vi "GVmotor_get_Alarm.vi"(8 "error in (no error)":errorcluster, 10 "milliseconds to wait":u32=100, 11 "VISA resource name":refnum<visa-resource-name>) -> (0 "error out":errorcluster, 2 "Alarm Code":i32, 3 "VISA resource name out":refnum<visa-resource-name>)   [LabVIEW 2019]
panel:
  out "trimmed string":string
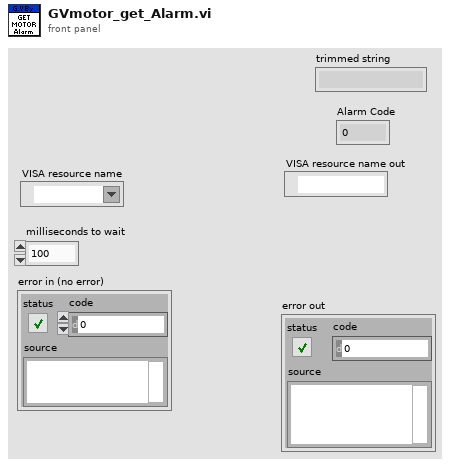
[diagram p1: front panel]
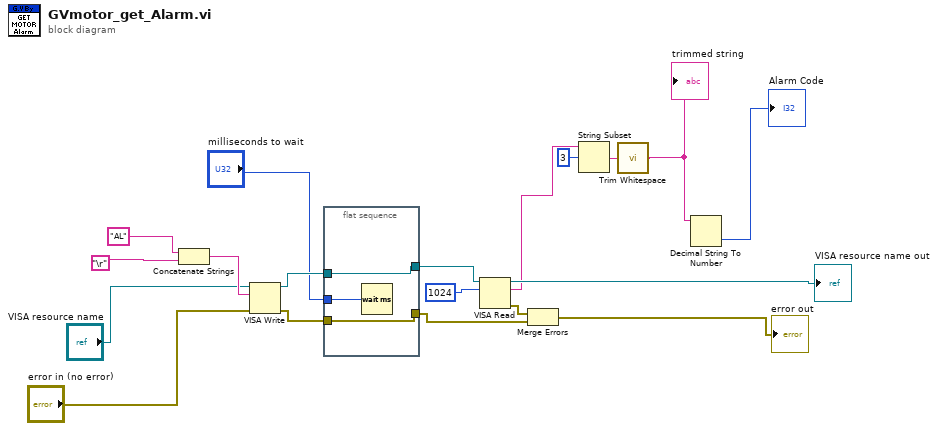
[diagram p0: block diagram]
diagram:
  n1 = Concatenate Strings("AL" ("string"), "\r") -> (w19:string)
  n2 = VISA Write(VISA resource name="VISA resource name", write buffer=w19, error in (no error)="error in (no error)") -> (VISA resource name out=w15:refnum<visa-resource-name>, error out=w16:errorcluster)  [unwired: 1 out]
  n3 = flat-sequence {
    tunnel: [w22] -> w10
    tunnel: w16 -> [w22]
    tunnel: [w21] -> w14
    tunnel: w15 -> [w21]
    tunnel: "milliseconds to wait" -> [w20]
    frame #0 {
      n4 = Wait (ms)(milliseconds to wait=w20) -> ()  [unwired: 1 out]
    }
  }
  n5 = VISA Read(VISA resource name=w14, byte count=u32 1024) -> (VISA resource name out=→"VISA resource name out":refnum<visa-resource-name>, read buffer=w5:string, error out=w9:errorcluster)  [unwired: 1 in, 1 out]
  n6 = Merge Errors(w9, w10) -> (→"error out":errorcluster)
  n7 = String Subset(string=w5, offset (0)=3) -> (substring=w3:string)  [unwired: 1 in]
  n8 = call <vilib>:"Trim Whitespace.vi"("string"=w3) -> ("trimmed string"=w2:string)  [unwired: 1 in]
  "trimmed string" <- w2
  n9 = Decimal String To Number(string=w2) -> (number=→"Alarm Code":i32)  [unwired: 2 in, 1 out]
